vi "MotorSubVI.vi"(9 "Stop Button":bool, 10 "Frequency [Hz]":dbl=1000.0, 11 "Slide":dbl(slide)=0.4 scale=0.0..1.0) -> (0 "error out":errorcluster, 3 "Duty Cycle":dbl=0.10119047619047619)   [LabVIEW 2019]
uses:
  <vilib>/myRIO/Instrument Drivers/Onboard IO/PWM/typedefs/PWM Reference.ctl
  <vilib>/myRIO/Common/Instrument Driver Framework/Utilities/typedefs/myRIO Generic Hardware Reference.ctl
  <vilib>/myRIO/Common/Instrument Driver Framework/Utilities/typedefs/Hardware Version Enum.ctl
  <vilib>/myRIO/Common/Instrument Driver Framework/Utilities/typedefs/myRIO v1.0 Reference.ctl
  <vilib>/myRIO/Common/Instrument Driver Framework/Utilities/typedefs/Generic FPGA Reference.ctl
  <vilib>/myRIO/Common/Instrument Driver Framework/myRIO v1.0/PWM/typedefs/PWM Channels Enum.ctl
  <vilib>/myRIO/Instrument Drivers/Onboard IO/PWM/typedefs/PWM Configuration.ctl
  <vilib>/userDefined/High Color/nirio_resource_hc.ctl
  <vilib>/myRIO/Common/Instrument Driver Framework/Utilities/vis/Is FPGA Ref Available.vi
  <vilib>/myRIO/Common/Instrument Driver Framework/myRIO v1.0/PWM/vis/myRIO v1.1 Open PWM.vi
  <vilib>/myRIO/Instrument Drivers/Onboard IO/PWM/vis/Set Duty Cycle and Frequency.vi
  <vilib>/myRIO/Common/Instrument Driver Framework/Utilities/vis/Validate Channels.vi
  <vilib>/myRIO/Common/Instrument Driver Framework/myRIO v1.0/PWM/vis/myRIO v1.0 Reserve PWM.vi
  <vilib>/myRIO/Common/Instrument Driver Framework/myRIO v1.0/UART/vis/myRIO v1.0 Close UART.vi
  <vilib>/myRIO/Common/Instrument Driver Framework/myRIO v1.0/PWM/vis/myRIO v1.0 Build MUX Configuration PWM.vi
  <vilib>/myRIO/Common/Instrument Driver Framework/myRIO v1.0/Resource Manager/vis/myRIO v1.0 Reserve Channel List.vi
  <vilib>/myRIO/Common/Instrument Driver Framework/myRIO v1.0/Resource Manager/vis/myRIO v1.0 Create Configuration List.vi
  <vilib>/myRIO/Common/Instrument Driver Framework/myRIO v1.0/Resource Manager/vis/myRIO v1.0 Reserve Channel.vi
  <vilib>/myRIO/Common/Instrument Driver Framework/myRIO v1.0/Resource Manager/vis/myRIO v1.0 Unreserve Channel.vi
  <vilib>/myRIO/Common/Instrument Driver Framework/myRIO v1.0/Resource Manager/vis/myRIO v1.0 Build Mutex Name.vi
  <vilib>/Utility/VariantDataType/GetNumericInfo.vi
  <vilib>/Utility/error.llb/Error Cluster From Error Code.vi
  <vilib>/myRIO/Common/Instrument Driver Framework/myRIO v1.0/myRIO v1.1 Open.vi
  <vilib>/myRIO/Common/Instrument Driver Framework/Utilities/vis/IO Manager.vi
  <vilib>/myRIO/Common/Instrument Driver Framework/Utilities/vis/Configuration Manager.vi
  <vilib>/myRIO/Common/Instrument Driver Framework/myRIO v1.0/Resource Manager/vis/myRIO v1.0 Configure IO.vi
  <vilib>/myRIO/Common/Instrument Driver Framework/myRIO v1.0/myRIO v1.0 Close.vi
  <vilib>/myRIO/Common/Instrument Driver Framework/myRIO v1.0/PWM/vis/myRIO v1.0 Write PWM.vi
  <vilib>/myRIO/Common/Instrument Driver Framework/Utilities/vis/FPGA Ref Manager.vi
  <vilib>/myRIO/Common/Instrument Driver Framework/myRIO v1.0/myRIO v1.0 Reset FPGA.vi
  <vilib>/myRIO/Common/Instrument Driver Framework/myRIO v1.0/IRQ/vis/myRIO v1.0 IRQ Info FGV.vi
  <vilib>/myRIO/Common/Instrument Driver Framework/myRIO v1.0/IRQ/vis/myRIO v1.0 Timer IRQ Info FGV.vi
  <vilib>/myRIO/Common/Instrument Driver Framework/myRIO v1.0/IRQ/vis/myRIO v1.0 ISR Agent.vi
  <vilib>/myRIO/Instrument Drivers/Utilities/vis/Reset Index.vi
  <vilib>/myRIO/Common/Instrument Driver Framework/myRIO v1.0/Resource Manager/vis/myRIO v1.0 Block Write Resource Manager.vi
  <vilib>/myRIO/Express VI/Onboard IO/PWM/PWM Express VI.xnode
  <vilib>/myRIO/Instrument Drivers/Onboard IO/PWM/vis/myRIO PWM Open.xnode
  <vilib>/myRIO/Instrument Drivers/Onboard IO/PWM/PWM.lvlib
  <vilib>/myRIO/Instrument Drivers/Utilities/Utilities.lvlib
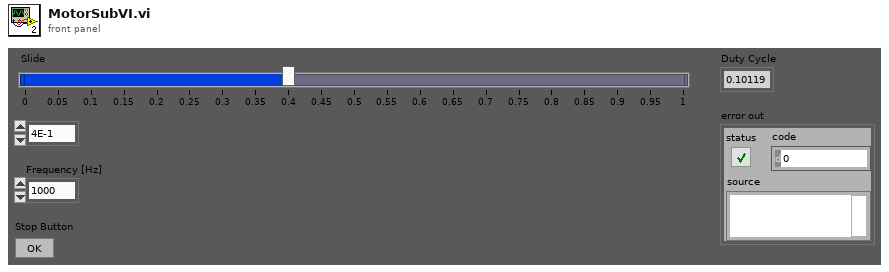
[diagram p1: front panel]
types:
  T1 = typedef "PWM.lvlib/PWM Reference.ctl" = cluster{"myRIO Reference":T2, "PWM Channels Enum":T6, "PWM Configuration":T7}
  T2 = typedef "myRIO Generic Hardware Reference.ctl" = cluster{"myRIO Model":T3, "myRIO Hardware Reference":T4}
  T3 = typedef "Hardware Version Enum.ctl" = enum16{"Unknown", "myRIO-1900", "myRIO-1950", "roboRIO", "NI ELVIS RIO CM", "ELVIS III"}
  T4 = typedef "myRIO v1.0 Reference.ctl" = cluster{"Generic FPGA Reference":T5, "Allow multiple opens":bool}
  T5 = typedef "Generic FPGA Reference.ctl" = refnum<k20>
  T6 = typedef "PWM Channels Enum.ctl" = enum16{"Not Connected", "C/PWM0", "C/PWM1", "A/PWM0", "A/PWM1", "A/PWM2", "A/PWM3", "A/PWM4", "A/PWM5", "A/PWM6", "A/PWM7", "A/PWM8", "A/PWM9", "A/PWM10", "A/PWM11", "A/PWM12", "A/PWM13", "A/PWM14", "A/PWM15", "A/PWM16", "A/PWM17", "A/PWM18", "A/PWM19", "B/PWM0", "B/PWM1", "B/PWM2", "B/PWM3", "B/PWM4", "B/PWM5", "B/PWM6", "B/PWM7", "B/PWM8", "B/PWM9", "B/PWM10", "B/PWM11", "B/PWM12", "B/PWM13", "B/PWM14", "B/PWM15", "B/PWM16", "B/PWM17", "B/PWM18", "B/PWM19", "PWM/PWM0", "PWM/PWM1", "PWM/PWM2", "PWM/PWM3", "PWM/PWM4", "PWM/PWM5", "PWM/PWM6", "PWM/PWM7", "PWM/PWM8", "PWM/PWM9"}
  T7 = typedef "PWM.lvlib/PWM Configuration.ctl" = cluster{"Frequency":dbl, "Duty Cycle":dbl}
  T8 = typedef "nirio_resource_hc.ctl" = tag
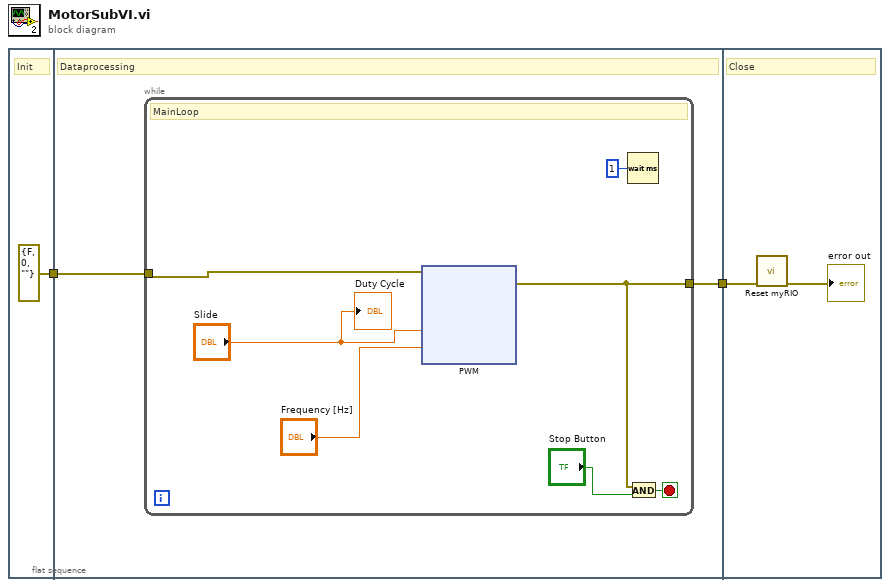
[diagram p0: block diagram]
diagram:
  n1 = flat-sequence {
    tunnel: [errorcluster {"status"=FALSE, "code"=0, "source"=""} ("error constant")] -> w2
    tunnel: w2 -> [w5]
    tunnel: [w4] -> w1
    tunnel: w1 -> [w48]
    frame #0 {
      # "Init"
    }
    frame #1 {
      # "Dataprocessing"
      n2 = while "Main Loop" {
        tunnel: w5 -> [w6]
        tunnel: [w7] -> w4
        stop <- w12 stop-if-true
        # "MainLoop"
        n3 = xnode "PWM"("Duty Cycle"="Slide", "Frequency [Hz]"="Frequency [Hz]", "error in (no error)"=w6) -> ("error out"=w7:errorcluster)
        n4 = Wait (ms)(milliseconds to wait=u32 1) -> ()  [unwired: 1 out]
        n5 = And(x=w7, y="Stop Button") -> (x .and. y?=w12:bool)
        "Duty Cycle" <- "Slide"
      }
    }
    frame #2 {
      # "Close"
      n6 = call <vilib>:"Reset myRIO.vi"("error in (no error)"=w48) -> ("error out"=→"error out":errorcluster)  [unwired: 10 in]
    }
  }
